vi "5HC.vi"() -> (0 "DAQ Error":errorcluster)   [LabVIEW 2020]
doc: "Use this plug-in with the Nathan 7609 data acquisition system"
uses:
  Globals/Meas_global.vi
  Globals/Dynamic_call_global.ph.vi
  Globals/Trav_pos_global.vi
  Globals/Extra_Commands_Global.vi
  Sub_vis/Upload Data.ctl
panel:
  # "Do not close this window between blocks"
  # "PN 06/06/18"
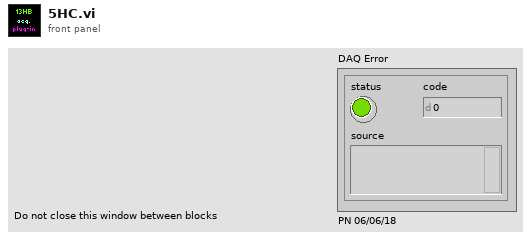
[diagram p1: front panel]
types:
  T1 = typedef "Analysis_info_cluster.ctl" = cluster{"Colour":u32, "Inst type":T2, "Inst name":string, "Symbol":string, "Code name":string, "Extra Info":string, "Inst Array":T3, "Extra Titles":string[], "Extra Values":string[], "U":dbl, "u^2":dbl, "u^3":dbl, "u^4":dbl, "Skew_u":dbl, "Kurt_u":dbl, "Sd Error in Mean":dbl, "% u'/U":dbl, "X":dbl, "Y":dbl, "Z":dbl, "Timescale integral Estimate":dbl, "Sd Error in Variance":dbl, "Calib File":path, "Calib Constants":dbl[], "Output Position":bool, "Stats":enum16{"None", "Basic", "Full"}, "Av Sampling Rate":dbl, "Av No of Samples":dbl, "Total Meas Time (s)":dbl, "ADAM Ch Name":string, "Max value":dbl, "Min value":dbl, "Req Sample Rate Hz":dbl, "Sync Delay Time (s)":dbl, "Ch No":i16, "Device":string, "Use Latest Calib":bool, "Port":string, "Metadata Ch Names":string[], "Metadata Ch Values":string[], "Label":string}
  T2 = typedef "Inst_type.ctl" = enum16{"Raw voltage", "Raw with zero offsetting", "Propeller anemometer", "Pressure Transducer", "Pitot-static tube", "Hot wire", "Cross wire 1", "Cross wire 2", "Generic Linear", "Generic Polynomial", "Generic BackPoly", "Fast FID", "Thermocouple", "Cold wire", "Pulsed Wire", "LDA Vel", "LDA Tran time", "LDA Arr time", "Microphone"}
  T3 = typedef "Instrument_Array.ctl" = enum16{"PWA", "LDA", "Analogue"}
  T4 = typedef "Device ID port info.ctl" = cluster{"Ch No":i16[], "Req Sampling Rate":dbl[], "Port":string, "Index":i32[]}
  T5 = typedef "Traverse_cluster.ctl" = cluster{"Start X":sgl, "Start Y":sgl, "Start Z":sgl, "End X":sgl, "End Y":sgl, "End Z":sgl, "No. of pts.":i32, "Spacing":T6, "Filename":path, "Tunnel Speed":dbl, "Averaging time (mins)":dbl, "Extra Commands":string, "Carrier_1 Q (l/min)":dbl, "Carrier_2 Q (l/min)":dbl, "Trace Gas Concentration (%)":dbl, "Specific Arguments":string, "Comments":string, "Row No":i32, "Row Type Selector":T7, "EstCompl":string, "Row Duration (mins)":dbl, "No. of Valid pts.":i32, "Meas Setup File":string}
  T6 = typedef "Spacing.ctl" = enum16{"Linear", "Log", "Gauss", "Specified", "N/A"}
  T7 = typedef "Multi_run_mode.ctl" = enum16{"Move Traverse Only", "Set Tunnel Speed Only", "Set Source Only", "Set Measurement Conditions", "Single Measurement", "Vertical Profile", "Lateral Profile", "Longitudinal Profile", "Multi-Axis Profile", "Explore Volume", "Auto Calibrate", "Meas Fast FID Bkgnd", "Check Beam Power", "Scanning Valve Measurement", "Run VI Named:", "Set ADAM Ch", "Wait (minutes)", "Send Message", "Synchronize With:", "Fall Back to this Row", "Turn Off Row Repeating", "Traverse 3D Volume", "Blank Row", "Jump to Fall Back Row"}
  T8 = typedef "Trigger_Mode.ctl" = enum16{"Free Running", "Start on Trigger", "Trigger Every Block", "Trigger Every Sample"}
  T9 = typedef "Upload Data.ctl" = enum16{"Voltage Array", "Time Trace Cluster"}
  T10 = typedef "Rendezvous RefNum" = refnum<k1>
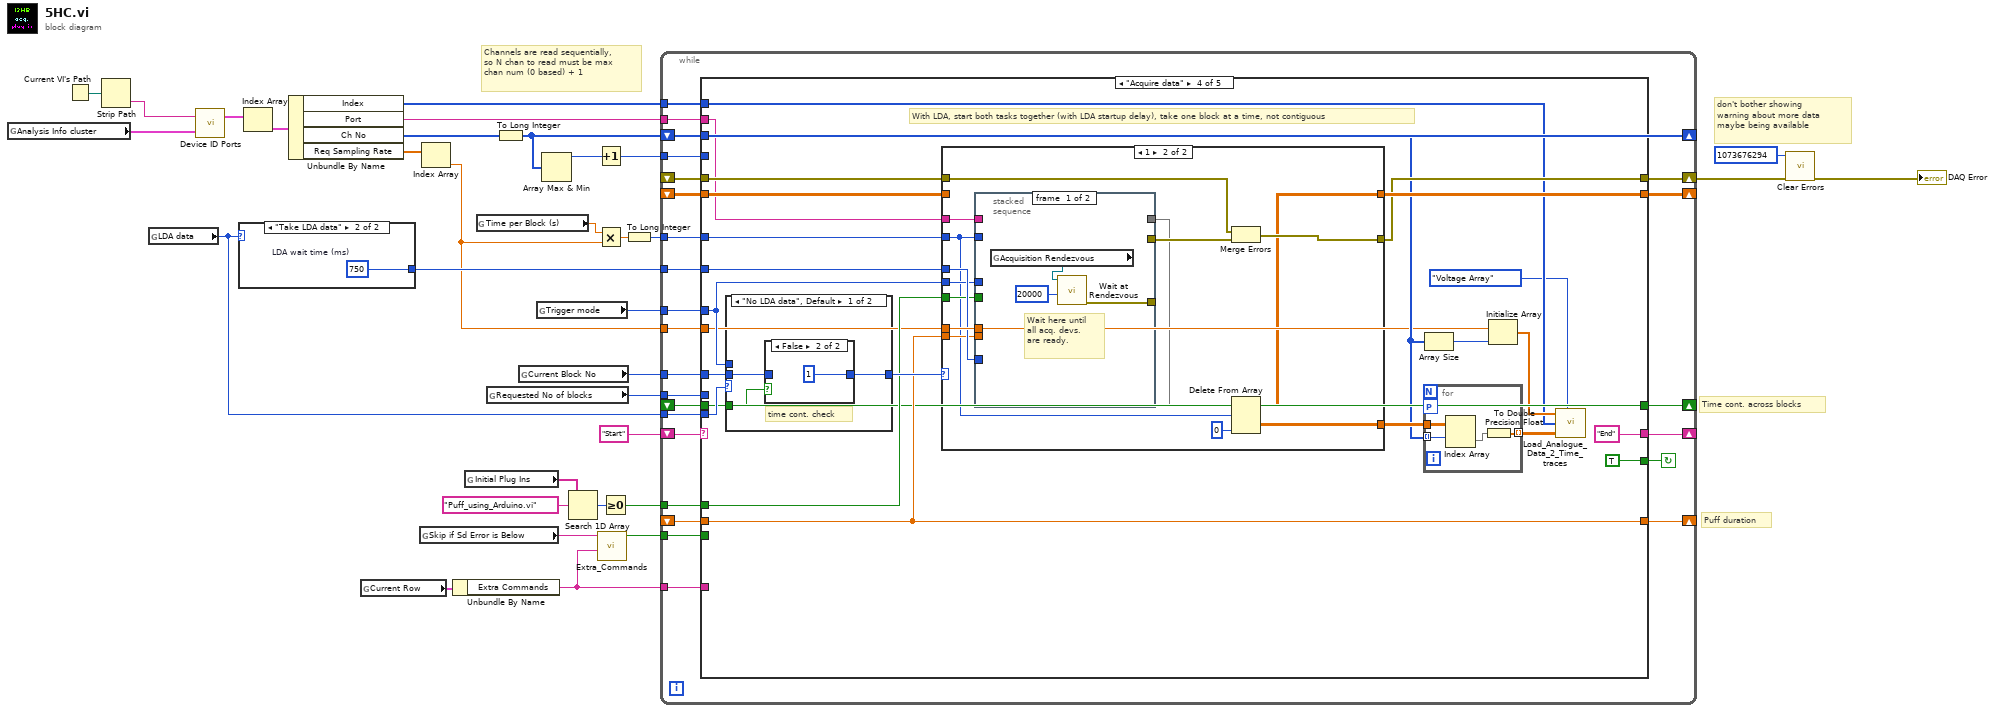
[diagram p0: block diagram]
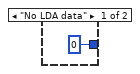
[diagram p2: hidden frame]
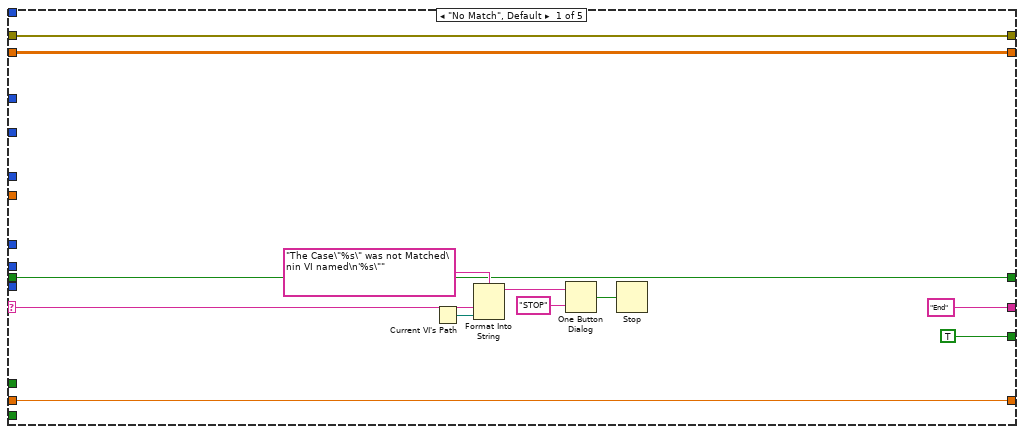
[diagram p3: hidden frame]
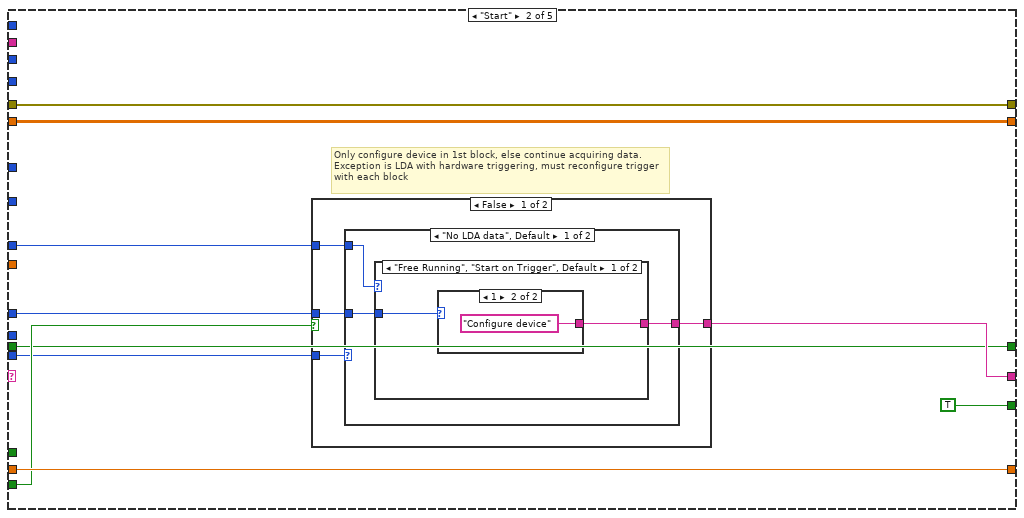
[diagram p4: hidden frame]
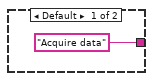
[diagram p5: hidden frame]
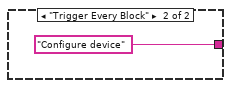
[diagram p6: hidden frame]
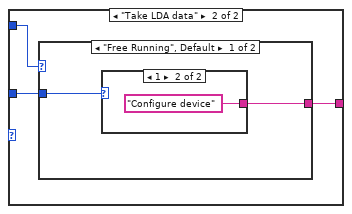
[diagram p7: hidden frame]
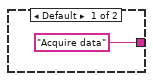
[diagram p8: hidden frame]
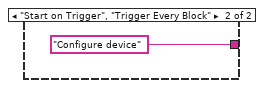
[diagram p9: hidden frame]
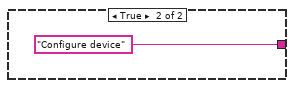
[diagram p10: hidden frame]
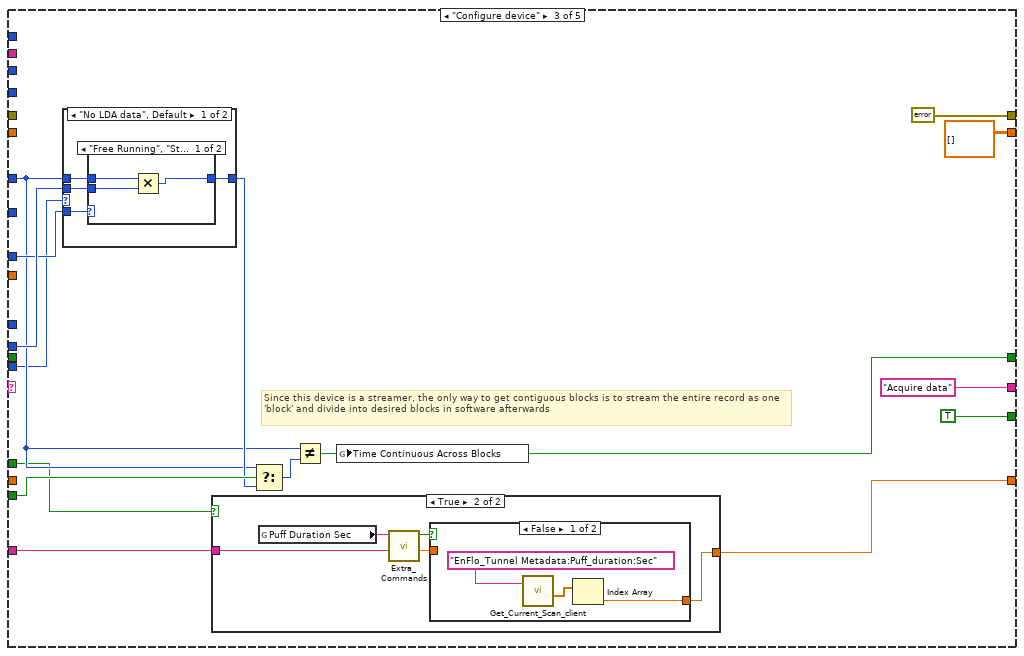
[diagram p11: hidden frame]
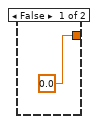
[diagram p12: hidden frame]
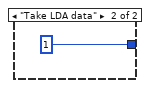
[diagram p17: hidden frame]
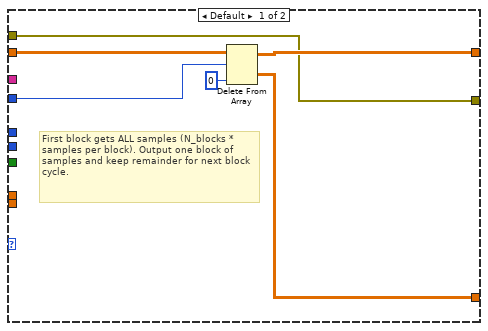
[diagram p18: hidden frame]
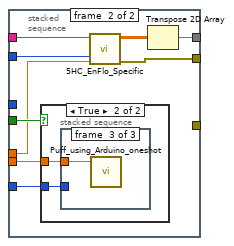
[diagram p19: hidden frame]
diagram:
  # "don't bother showing warning about more data maybe being available"
  # "Time cont. across blocks"
  # "Puff duration"
  # "Channels are read sequentially, so N chan to read must be max chan num (0 based) + 1"
  n1 = global read "Meas_global.vi" "Analysis Info cluster"() -> (w3:T1[])
  n2 = Current VI's Path() -> (path=w11:path)
  n3 = Strip Path(path=w11) -> (name=w2:string)  [unwired: 1 out]
  n4 = global read "Meas_global.vi" "LDA data"() -> (w30:enum16{"No LDA data", "Take LDA data"})
  n5 = call "Device ID Ports.vi"("Analysis Info cluster"=w3, "Device ID"=w2) -> ("Device port info"=w9:T4[])  [unwired: 1 out]
  n6 = case shown="\"Take LDA data\"" w30 {
    tunnel: [u32 0 ("LDA wait time (ms)") w35] -> w25
    frame "No LDA data" {
    }
    frame "Take LDA data" {
      w35 = u32 750  # LDA wait time (ms)
    }
  }
  n7 = Index Array(array=w9) -> (element=w8:T4)  [unwired: 1 in]
  n8 = Unbundle By Name(w8) -> ("Index"=w7:i32[], "Port"=w6:string, "Ch No"=w5:i16[], "Req Sampling Rate"=w4:dbl[])
  n9 = global read "Trav_pos_global.vi" "Current Row"() -> (w19:T5)
  n10 = global read "Extra_Commands_Global.vi" "Skip if Sd Error is Below"() -> (w18:string)
  n11 = Index Array(array=w4) -> (element=w10:dbl)  [unwired: 1 in]
  n12 = Unbundle By Name(w19) -> ("Extra Commands"=w17:string)
  n13 = global read "Dynamic_call_global.ph.vi" "Initial Plug Ins"() -> (w27:string[])
  n14 = global read "Meas_global.vi" "Time per Block (s)"() -> (w13:dbl)
  n15 = global read "Meas_global.vi" "Requested No of blocks"() -> (w24:i32)
  n16 = To Long Integer(number=w5) -> (32bit integer=w22:i32[])
  n17 = global read "Meas_global.vi" "Current Block No"() -> (w31:i32)
  n18 = global read "Meas_global.vi" "Trigger mode"() -> (w32:T8)
  n19 = Array Max & Min(array=w22) -> (max value=w21:i32)  [unwired: 3 out]
  n20 = Search 1D Array(1D array=w27, element="Puff_using_Arduino.vi") -> (index of element=w29:i32)  [unwired: 1 in]
  n21 = Increment(x=w21) -> (x+1=w20:i32)
  n22 = Multiply(x=w13, y=w10) -> (x*y=w12:dbl)
  n23 = call "Extra_Commands.vi"("String to Search"=w17, "Command"=w18) -> ("Command Found"=w16:bool)  [unwired: 2 in, 3 out]
  n24 = Greater Or Equal To 0?(x=w29) -> (x >= 0?=w26:bool)
  n25 = To Long Integer(number=w12) -> (32bit integer=w23:i32)
  n26 = while {
    shift-left: "Start" -> [w60]
    shift-right: [w48] -> _
    tunnel: w10 -> [w59]
    tunnel: w23 -> [w58]
    tunnel: w31 -> [w57]
    tunnel: w32 -> [w55]
    tunnel: w30 -> [w54]
    tunnel: w24 -> [w53]
    shift-right: [w51] -> w1
    shift-left: _ -> [w52]
    shift-right: [w50] -> _
    shift-left: _ -> [w49]
    tunnel: w25 -> [w47]
    tunnel: w26 -> [w46]
    shift-right: [w45] -> _
    shift-left: _ -> [w44]
    shift-right: [w43] -> _
    shift-left: w22 -> [w43]
    tunnel: w20 -> [w42]
    tunnel: w17 -> [w41]
    tunnel: w16 -> [w40]
    shift-right: [w39] -> _
    shift-left: _ -> [w38]
    tunnel: w6 -> [w37]
    tunnel: w7 -> [w36]
    stop <- w56 continue-if-true
    n27 = case shown="\"Acquire data\"" w60 {
      selector: w60 -> [w65 _ _ _ _]
      tunnel: ["End" w79 "Acquire data" ("f") "End" "End" ("f")] -> w48
      tunnel: w59 -> [_ _ _ w140 _]
      tunnel: w58 -> [_ _ w109 w158 _]
      tunnel: w57 -> [_ w80 _ w154 _]
      tunnel: [TRUE TRUE TRUE TRUE FALSE] -> w56
      tunnel: w55 -> [_ w73 w114 w149 _]
      tunnel: w54 -> [_ w74 w106 w152 _]
      tunnel: w53 -> [_ _ w117 _ _]
      tunnel: w52 -> [w64 w81 _ w159 w208]
      tunnel: [w64 w81 errorcluster {"status"=FALSE, "code"=0, "source"=""} ("error IO") w146 w208] -> w51
      tunnel: [w63 w78 sgl[][] [] ("Channel volts") w156 w211] -> w50
      tunnel: w49 -> [w63 w78 _ w157 w211]
      tunnel: w47 -> [_ _ _ w153 _]
      tunnel: w46 -> [_ _ w105 w151 _]
      tunnel: [w62 w77 w113 w150 w210] -> w45
      tunnel: w44 -> [w62 w77 _ w150 w210]
      tunnel: w43 -> [_ _ _ w145 _]
      tunnel: w42 -> [_ _ _ _ _]
      tunnel: w41 -> [_ _ w112 _ _]
      tunnel: w40 -> [_ w76 w111 _ _]
      tunnel: [w61 w75 w107 w147 w209] -> w39
      tunnel: w38 -> [w61 w75 _ w147 w209]
      tunnel: w37 -> [_ _ _ w139 _]
      tunnel: w36 -> [_ _ _ w142 _]
      frame "No Match", Default {
        n28 = Current VI's Path() -> (path=w68:path)
        n29 = Format Into String(format string="The Case\"%s\" was not Matched\nin VI named\n'%s\"" ("Format String"), w65, w68) -> (resulting string=w71:string)  [unwired: 2 in, 1 out]
        n30 = One Button Dialog(message=w71, button name ("OK")="STOP") -> (true=w69:bool)
        n31 = Stop(stop? (T)=w69) -> ()
      }
      frame "Start" {
        # "Only configure device in 1st block, else continue acquiring data. Exception is LDA with hardware triggering, must reconfigure trigger with each block"
        n32 = case shown="False" w76 {
          tunnel: w80 -> [w86 _]
          tunnel: [w85 "Configure device" ("f")] -> w79
          tunnel: w74 -> [w84 _]
          tunnel: w73 -> [w83 _]
          frame False {
            n33 = case shown="\"No LDA data\", Default" w84 {
              tunnel: w86 -> [w89 w95]
              tunnel: [w88 w96] -> w85
              tunnel: w83 -> [w87 w97]
              frame "No LDA data", Default {
                n34 = case shown="\"Free Running\", \"Start on Trigger\", Default" w87 {
                  tunnel: w89 -> [w91 _]
                  tunnel: [w90 "Configure device" ("f")] -> w88
                  frame "Free Running", "Start on Trigger", Default {
                    n35 = case shown="1" w91 {
                      tunnel: ["Acquire data" ("f") "Configure device" ("f")] -> w90
                      frame Default {
                      }
                      frame 1 {
                      }
                    }
                  }
                  frame "Trigger Every Block" {
                  }
                }
              }
              frame "Take LDA data" {
                n36 = case shown="\"Free Running\", Default" w97 {
                  tunnel: [w99 "Configure device" ("f")] -> w96
                  tunnel: w95 -> [w98 _]
                  frame "Free Running", Default {
                    n37 = case shown="1" w98 {
                      tunnel: ["Acquire data" ("f") "Configure device" ("f")] -> w99
                      frame Default {
                      }
                      frame 1 {
                      }
                    }
                  }
                  frame "Start on Trigger", "Trigger Every Block" {
                  }
                }
              }
            }
          }
          frame True {
          }
        }
      }
      frame "Configure device" {
        # "Since this device is a streamer, the only way to get contiguous blocks is to stream the entire record as one 'block' and divide into desired blocks in software afterwards"
        n38 = case shown="\"No LDA data\", Default" w106 {
          tunnel: [w130 w137] -> w110
          tunnel: w109 -> [w132 w137]
          tunnel: w117 -> [w131 _]
          tunnel: w114 -> [w129 _]
          frame "No LDA data", Default {
            n39 = case shown="\"Free Running\", \"Start on Trigger\", Default" w129 {
              tunnel: w132 -> [w135 w136]
              tunnel: w131 -> [w134 _]
              tunnel: [w133 w136] -> w130
              frame "Free Running", "Start on Trigger", Default {
                n40 = Multiply(x=w135, y=w134) -> (x*y=w133:i32)
              }
              frame "Trigger Every Block" {
              }
            }
          }
          frame "Take LDA data" {
          }
        }
        n41 = case shown="True" w105 {
          tunnel: [0.0 w124] -> w113
          tunnel: w112 -> [_ w120]
          frame False {
          }
          frame True {
            n42 = global read "Extra_Commands_Global.vi" "Puff Duration Sec"() -> (w123:string)
            n43 = call "Extra_Commands.vi"("String to Search"=w120, "Command"=w123) -> ("Numeric Value"=w121:dbl, "Command Found"=w122:bool)  [unwired: 2 in, 2 out]
            n44 = case shown="False" w122 {
              tunnel: [w126 w128] -> w124
              tunnel: w121 -> [_ w128]
              frame False {
                n45 = call "Get_Current_Scan_client.vi"("singleChannel"="EnFlo_Tunnel Metadata:Puff_duration:Sec") -> ("Numerical Values"=w127:dbl[])  [unwired: 1 in, 3 out]
                n46 = Index Array(array=w127) -> (element=w126:dbl)  [unwired: 1 in]
              }
              frame True {
              }
            }
          }
        }
        n47 = Select(t=w109, s=w111, f=w110) -> (s? t:f=w108:i32)
        n48 = Not Equal?(x=w109, y=w108) -> (x != y?=w107:bool)
        n49 = global write "Meas_global.vi" "Time Continuous Across Blocks"(w107) -> ()
      }
      frame "Acquire data" {
        # "With LDA, start both tasks together (with LDA startup delay), take one block at a time, not contiguous"
        n50 = case shown="\"No LDA data\", Default" w152 {
          tunnel: w154 -> [w167 _]
          tunnel: w149 -> [_ _]
          tunnel: [w168 1 ("Current Block No")] -> w155
          tunnel: w147 -> [w166 _]
          frame "No LDA data", Default {
            # "time cont. check"
            n51 = case shown="False" w166 {
              tunnel: [w169 1 ("Current Block No")] -> w168
              tunnel: w167 -> [w169 _]
              frame True {
              }
              frame False {
              }
            }
          }
          frame "Take LDA data" {
          }
        }
        n52 = case shown="1" w155 {
          tunnel: w159 -> [w173 w190]
          tunnel: [w173 w189] -> w146
          tunnel: [w175 w188] -> w156
          tunnel: w158 -> [w174 w179]
          tunnel: w157 -> [w176 _]
          tunnel: [w172 w186] -> w148
          tunnel: w153 -> [_ w185]
          tunnel: w151 -> [_ w184]
          tunnel: w150 -> [_ w183]
          tunnel: w149 -> [_ w182]
          tunnel: w140 -> [_ w180]
          tunnel: w139 -> [_ w178]
          frame Default {
            # "First block gets ALL samples (N_blocks * samples per block). Output one block of samples and keep remainder for next block cycle."
            n53 = Delete From Array(array=w176, length=w174, index (col)=0 ("disabled index (col)")) -> (deleted portion=w172:sgl[][], array with subset deleted=w175:sgl[][])  [unwired: 1 in]
          }
          frame 1 {
            n54 = stacked-sequence {
              tunnel: [_ w195] -> w181
              tunnel: [_ w199] -> w191
              tunnel: w185 -> [_ w203]
              tunnel: w184 -> [_ w202]
              tunnel: w183 -> [_ w201]
              tunnel: w182 -> [_ _]
              tunnel: w180 -> [_ w198]
              tunnel: w179 -> [_ w197]
              tunnel: w178 -> [_ w196]
              tunnel: [w193 _] -> _
              frame #0 {
                # "Wait here until all acq. devs. are ready."
                n55 = global read "Meas_global.vi" "Acquisition Rendezvous"() -> (w194:T10)
                n56 = call <vilib>:"Wait at Rendezvous.vi"("ms timeout (-1)"=20000, "rendezvous"=w194) -> ("error out"=w193:errorcluster)  [unwired: 3 in, 2 out]
              }
              frame #1 {
                n57 = case shown="True" w202 {
                  tunnel: w201 -> [_ w205]
                  tunnel: w203 -> [_ w204]
                  frame False {
                  }
                  frame True {
                    n58 = stacked-sequence {
                      tunnel: w205 -> [_ _ w207]
                      tunnel: w204 -> [_ w206 _]
                      frame #0 {
                      }
                      frame #1 {
                        n59 = Wait (ms)(milliseconds to wait=w206) -> ()  [unwired: 1 out]
                      }
                      frame #2 {
                        n60 = call "Puff_using_Arduino_oneshot.vi"("Puff_duration:Sec"=w207) -> ()  [unwired: 7 in]
                      }
                    }
                  }
                }
                n61 = call "5HC_EnFlo_Specific.vi"("Data rate (Hz)"=w198, "N samples"=w197, "COM Port"=w196) -> ("I/O error"=w199:errorcluster, "Data"=w200:sgl[][])  [unwired: 5 in, 2 out]
                n62 = Transpose 2D Array(2D array=w200) -> (transposed array=w195:sgl[][])
              }
            }
            n63 = Merge Errors(w190, w191) -> (w189:errorcluster)
            n64 = Delete From Array(array=w181, length=w179, index (col)=0 ("disabled index (col)")) -> (deleted portion=w186:sgl[][], array with subset deleted=w188:sgl[][])  [unwired: 1 in]
          }
        }
        n65 = for {
          tunnel: w145 -> [w164] mode=indexing
          workers-P: _ -> [_]
          tunnel: w148 -> [w165]
          tunnel: [w162] -> w141 mode=indexing
          n66 = Index Array(array=w165, index (row)=w164) -> (element=w163:sgl[])  [unwired: 1 in]
          n67 = To Double Precision Float(number=w163) -> (double precision float=w162:dbl[])
        }
        n68 = Array Size(array=w145) -> (size(s)=w144:i32)
        n69 = Initialize Array(w140, w144) -> (w143:dbl[])
        n70 = call "Load_Analogue_Data_2_Time_traces.vi"("Sampling Rate (Hz)"=w143, "Mode"=Upload_Data."Voltage Array", "Index"=w142, "Voltage Array"=w141) -> ()  [unwired: 3 in]
      }
      frame "End" {
        n71 = global write "Meas_global.vi" "Acq ready"(FALSE ("Acq ready")) -> ()
      }
    }
  }
  n72 = call <vilib>:"Clear Errors.vi"("error in (no error)"=w1, "specific error code to clear (0: all)"=1073676294) -> ("error out"=→"DAQ Error":errorcluster)  [unwired: 4 in, 1 out]
